vi "CreatePublicEvents.vi"(8 "error in (no error)":errorcluster, 11 "SMO.UI":refnum<class "SMO.UI.lvclass">) -> (0 "error out":errorcluster, 3 "SMO.UI out":refnum<class "SMO.UI.lvclass">)   [LabVIEW 2021, in "smo.lvlib" / "SMO.UI.lvclass"]
uses:
  SMO.UI.lvclass
  Typedefs/SMO.UI State--enum.ctl
  SMO.UI.lvclass/SMO.UI.ctl
  SMO/SMO.lvclass
panel:
  # "For instructions on how to use the JKI State Machine Objects, examples and video tutorials, visit:\nhttp://jki.net/state-machine-objects/\n\nJKI State Machine Objects™\nhttp://jki.net/state-machine-objects/\nCopyright (C) 2005-2015, JKI <info@jki.net>\nALL RIGHTS RESERVED"
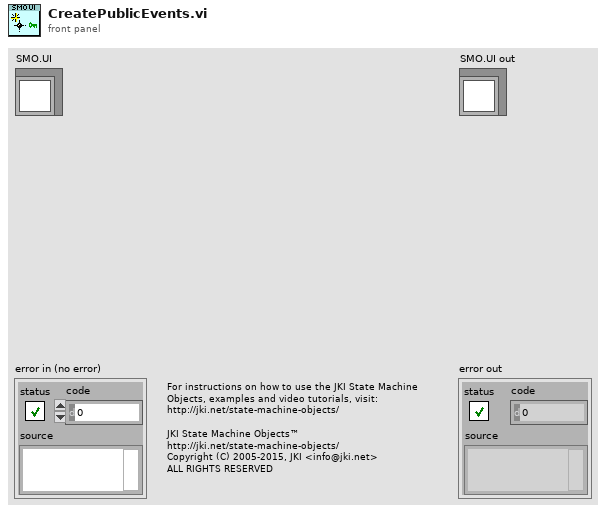
[diagram p1: front panel]
types:
  T1 = typedef "smo.lvlib/SMO.UI.lvclass/SMO.UI State--enum.ctl" = enum16{"unknown", "Opened", "Closed"}
  T2 = typedef "smo.lvlib/SMO.UI.lvclass/PrivateData--Ref.ctl" = refnum<data-value>
  T3 = cluster{"UI Closed":refnum<user-event>, "UI State":refnum<user-event>}
  T4 = typedef "smo.lvlib/SMO.UI.lvclass/PrivateData--Cluster.ctl" = cluster{"Public Events":T5, "Private Events":T6}
  T5 = typedef "smo.lvlib/SMO.UI.lvclass/PublicEvents--Cluster.ctl" = cluster{"UI Hidden":refnum<user-event>, "UI State":refnum<user-event>}
  T6 = typedef "smo.lvlib/SMO.UI.lvclass/PrivateEvents--Cluster.ctl" = cluster{"Show-Hide UI":refnum<user-event>}
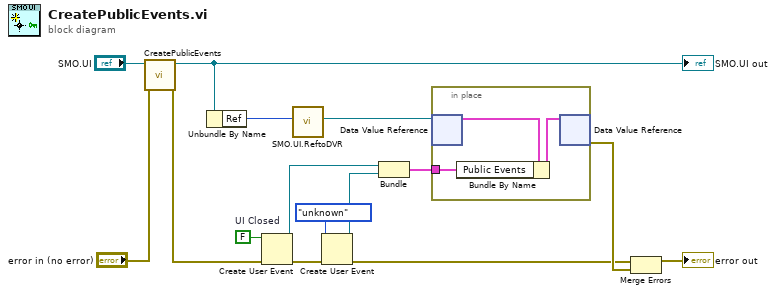
[diagram p0: block diagram]
diagram:
  w7 = FALSE  # UI Closed
  n1 = call-parent "CreatePublicEvents.vi"("error in (no error)"="error in (no error)", "SMO"="SMO.UI") -> ("error out"=w11:errorcluster, "SMO out"=w1:refnum<class "SMO.UI.lvclass">)  [unwired: 8 in]
  "SMO.UI out" <- w1
  n2 = Unbundle By Name(w1) -> ("Ref"=w9:u32)
  n3 = Create User Event(user event datatype=w7, error in=w11) -> (user event=w5:refnum<user-event>, error out=w4:errorcluster)
  n4 = call "SMO.UI.ReftoDVR.vi"("Ref"=w9) -> ("Ref"=w8:T2)  [unwired: 10 in]
  n5 = Create User Event(user event datatype=SMO.UI_State--enum."unknown" ("UI State"), error in=w4) -> (user event=w3:refnum<user-event>, error out=w10:errorcluster)
  n6 = Bundle("UI Closed"=w5, "UI State"=w3) -> (w6:T3)  [unwired: 1 in]
  n7 = in-place {
    in-place-border: w6 -> [w16]
    n8 = in-place-dvr #1(w8) -> (w18:T4)  [unwired: 1 out]
    n9 = Bundle By Name(cluster=w18, "Public Events"=w16) -> (w17:T4)
    n10 = in-place-dvr #1(w17) -> (w15:errorcluster)  [unwired: 1 out]
  }
  n11 = Merge Errors(w10, w15) -> (→"error out":errorcluster)
